vi "numap_tcp.vi"() -> ()   [LabVIEW 2024]
panel:
  out "错误输出":errorcluster
  out "W":dbl
  in  "加热功率":dbl(slide) scale=100.0..5000.0
  out "MPa":dbl
  in  "入口压力":dbl(slide) scale=8.0..12.0
  out "℃":dbl
  in  "入口温度":dbl(slide) scale=10.0..30.0 scale format="%#.6g"
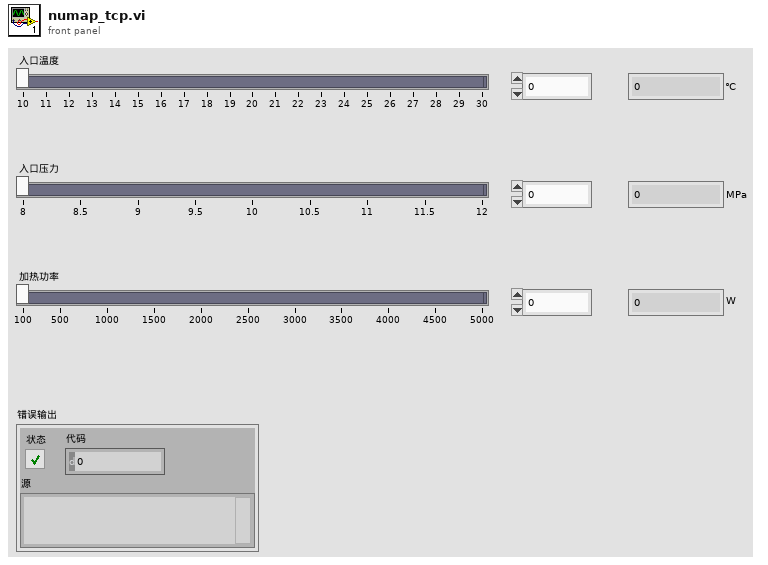
[diagram p1: front panel]
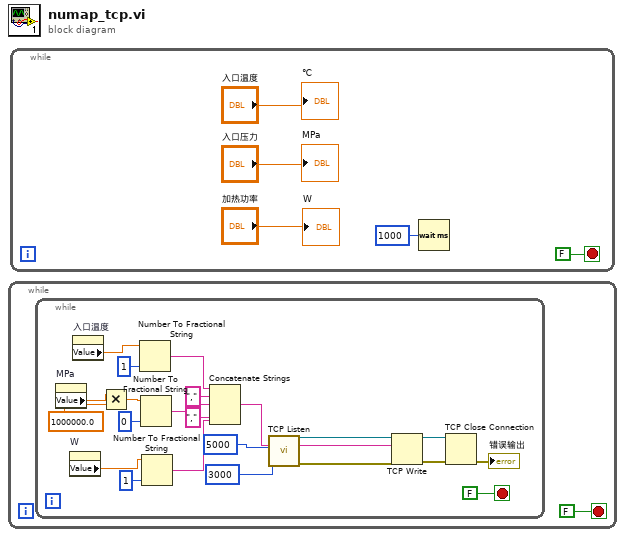
[diagram p0: block diagram]
diagram:
  n1 = while {
    stop <- FALSE stop-if-true
    n2 = while {
      stop <- FALSE stop-if-true
      n3 = property on="MPa" class="DigNum (严格)"() -> ("Value"=w4:dbl)  [unwired: 2 in, 2 out]
      n4 = property on="W" class="DigNum (严格)"() -> ("Value"=w5:dbl)  [unwired: 2 in, 2 out]
      n5 = property on="入口温度" class="Slide (严格)"() -> ("Value"=w6:dbl)  [unwired: 2 in, 2 out]
      n6 = Multiply(x=w4, y=1000000.0) -> (x*y=w2:dbl)
      n7 = Number To Fractional String(number=w6, precision (6)=i16 1) -> (F-format string=w15:string)  [unwired: 2 in]
      n8 = Number To Fractional String(number=w2, precision (6)=i16 0) -> (F-format string=w13:string)  [unwired: 2 in]
      n9 = Number To Fractional String(number=w5, precision (6)=i16 1) -> (F-format string=w11:string)  [unwired: 2 in]
      n10 = Concatenate Strings(w15, "," ("字符串"), w13, "," ("字符串"), w11) -> (w10:string)
      n11 = call <vilib>:"TCP Listen.vi"("timeout ms (wait forever: -1)"=3000, "port"=u16 5000) -> ("error out"=w20:errorcluster, "connection ID"=w19:refnum<k5>)  [unwired: 5 in, 3 out]
      n12 = TCP Write(connection ID=w19, data in=w10, error in (no error)=w20) -> (connection ID out=w18:refnum<k5>, error out=w22:errorcluster)  [unwired: 1 in, 1 out]
      n13 = TCP Close Connection(connection ID=w18, error in (no error)=w22) -> (error out=→"错误输出":errorcluster)  [unwired: 1 in, 1 out]
    }
  }
  n14 = while {
    stop <- FALSE stop-if-true
    n15 = Wait (ms)(milliseconds to wait=u32 1000 ("等待时间（毫秒）")) -> ()  [unwired: 1 out]
    "℃" <- "入口温度"
    "MPa" <- "入口压力"
    "W" <- "加热功率"
  }
